vi "Window Plots.vi"() -> ()   [LabVIEW 2009]
uses:
  <vilib>/Analysis/4window.llb/Force Window (DBL).vi
  <vilib>/Analysis/4window.llb/Kaiser-Bessel Window (DBL).vi
  <vilib>/Analysis/4window.llb/Hamming Window (DBL).vi
  <vilib>/Analysis/4window.llb/Hanning Window (DBL).vi
  <vilib>/Analysis/4window.llb/Triangle Window (DBL).vi
  <vilib>/Analysis/4window.llb/Exponential Window (DBL).vi
  <vilib>/Analysis/NI_AALBase.lvlib
  <vilib>/Analysis/NI_AALPro.lvlib
panel:
  in  "beta (Kaiser-Bessel)":dbl=10.0 format="%.2f"
  in  "final value (exponential)":dbl=0.1 min=0.0 max=1.01 step=0.05 format="%.2f"
  out "Window":dbl[](graph)=[1.0, 0.9820327790631257, 0.9643883791544459, 0.9470610000772238, 0.9300449458481391, 0.9133346228248623, 0.8969245378672713, 0.8808092965317061, 0.8649836012976682, 0.8494422498263797, 0.8341801332506336, 0.8191922344953683, 0.8044736266284181, 0.7900194712408969, 0.775825016856679, 0.7618855973704608, 0.7481966305138833, 0.7347536163492154, 0.7215521357901017, 0.7085878491488874, 0.6958564947100447, 0.6833538873292304, 0.6710759170575142, 0.6590185477903263, 0.6471778159406794, 0.6355498291362295, 0.6241307649397461, 0.6129168695925733, 0.6019044567806661, 0.5910899064227986, 0.5804696634805439, 0.5700402367896358, 0.5597981979123283, 0.5497401800103734, 0.5398628767382501, 0.5301630411562773, 0.5206374846632573, 0.5112830759482941, 0.5020967399614464, 0.4930754569028748, 0.48421626123015066, 0.4755162406834013, 0.46697253532797073, 0.45858233661428077, 0.4503428864545839, 0.44225147631630474, 0.43430544633167084, 0.4265021844233419, 0.41883912544574825, 0.4113137503418573, 0.40392358531509076, 0.39666620101612016, 0.389539211744273, 0.38254027466328777, 0.37566708903115986, 0.3689173954438246, 0.3622889750924292, 0.3557796490339497, 0.3493872774749131, 0.3431097590679883, 0.336945030221216, 0.3308910644196496, 0.32494587155918425, 0.31910749729235516, 0.31337402238589035, 0.3077435620898061, 0.3022142655178378, 0.2967843150390036, 0.29145192568009887, 0.28621534453892705, 0.2810728502080725, 0.27602275220902706, 0.27106339043648336, 0.2661931346126128, 0.26141038375114883, 0.2567135656310988, 0.2521011362799121, 0.24757157946593383, 0.24312340619997844, 0.23875515424585797, 0.23446538763970512, 0.23025269621793265, 0.22611569515367402, 0.222053024501553, 0.21806334875063244, 0.21414535638539514, 0.21029775945461304, 0.20651929314796233, 0.20280871538024578, 0.19916480638308523, 0.19558636830395051, 0.19207222481239256, 0.1886212207133513, 0.18523222156741156, 0.1819041133178818, 0.17863580192457318, 0.17542621300415864, 0.17227429147699375, 0.1691790012202831, 0.16613932472747853, 0.1631542627737968, 0.16022283408774715, 0.15734407502856043, 0.15451703926941412, 0.1517407974863489, 0.14901443705277412, 0.14633706173946298, 0.14370779141993703, 0.14112576178114475, 0.1385901240393382, 0.1361000446610546, 0.13365470508911098, 0.13125330147352218, 0.12889504440725325, 0.12657915866671993, 0.12430488295695132, 0.12207146966133149, 0.1198781845958374, 0.11772430676769262, 0.11560912813835714, 0.11353195339077587, 0.1114920997008089, 0.10948889651276847, 0.10752168531898901, 0.10558981944335767, 0.10369266382873421, 0.10182959482819032, 0.09999999999999984]
  in  "stop":bool
  out "?":string="Exponential"
  out "Original Sine Wave":dbl[](graph)=[0.0, 0.47139673682599764, 0.8314696123025452, 0.9951847266721968, 0.9238795325112867, 0.6343932841636455, 0.19509032201612816, -0.29028467725446255, -0.7071067811865477, -0.9569403357322088, -0.9807852804032304, -0.7730104533627369, -0.38268343236508956, 0.09801714032956091, 0.5555702330196025, 0.8819212643483553, 1.0, 0.8819212643483552, 0.5555702330196023, 0.09801714032956063, -0.38268343236508984, -0.7730104533627371, -0.9807852804032305, -0.9569403357322087, -0.7071067811865472, -0.2902846772544619, 0.19509032201612886, 0.634393284163646, 0.9238795325112871, 0.9951847266721968, 0.8314696123025447, 0.4713967368259967, -1.1640536624890618e-15, -0.47139673682599875, -0.831469612302545, -0.9951847266721967, -0.9238795325112882, -0.6343932841636497, -0.1950903220161353, 0.2902846772544539, 0.70710678118654, 0.9569403357322053, 0.9807852804032332, 0.7730104533627469, 0.3826834323651057, -0.09801714032954173, -0.5555702330195851, -0.8819212643483445, -1.0, -0.8819212643483672, -0.5555702330196249, -0.09801714032958952, 0.38268343236506136, 0.7730104533627163, 0.9807852804032238, 0.9569403357322193, 0.707106781186574, 0.29028467725449986, -0.1950903220160882, -0.6343932841636126, -0.9238795325112699, -0.9951847266722014, -0.8314696123025717, -0.4713967368260411, -5.096259785702939e-14, 0.47139673682595123, 0.831469612302515, 0.9951847266721917, 0.9238795325113062, 0.6343932841636831, 0.19509032201617424, -0.2902846772544193, -0.707106781186517, -0.956940335732197, -0.9807852804032381, -0.7730104533627608, -0.3826834323651227, 0.09801714032952698, 0.5555702330195756, 0.8819212643483408, 1.0, 0.8819212643483675, 0.5555702330196225, 0.09801714032958306, -0.38268343236507063, -0.773010453362725, -0.9807852804032271, -0.9569403357322133, -0.7071067811865569, -0.29028467725447327, 0.19509032201611895, 0.6343932841636396, 0.9238795325112845, 0.9951847266721973, 0.8314696123025463, 0.4713967368259978, -1.715804148066935e-15, -0.4713967368260008, -0.8314696123025482, -0.9951847266721976, -0.9238795325112832, -0.6343932841636369, -0.1950903220161156, 0.29028467725447654, 0.7071067811865593, 0.9569403357322143, 0.9807852804032264, 0.7730104533627228, 0.38268343236506747, -0.09801714032958649, -0.5555702330196254, -0.881921264348369, -1.0, -0.8819212643483393, -0.5555702330195729, -0.09801714032952356, 0.38268343236512586, 0.773010453362763, 0.9807852804032388, 0.956940335732196, 0.7071067811865146, 0.29028467725441603, -0.1950903220161776, -0.6343932841636858, -0.9238795325113074, -0.9951847266721914, -0.8314696123025132, -0.4713967368259451]
  out "Windowed Sine Wave":dbl[](graph)=[0.0, 0.46292704750652336, 0.801859631724627, 0.9425006425037493, 0.8592494897846639, 0.5794133509142289, 0.1749812969166929, -0.25568544236643653, -0.6116357700927423, -0.8128655517339787, -0.8181515958970268, -0.6332441605784981, -0.3078587286853546, 0.0774354493757045, 0.43102528539750223, 0.6719231093217588, 0.7481966305138833, 0.6479948383152263, 0.4008728882166985, 0.06945375464584803, -0.2662927518291799, -0.5282396982515571, -0.6581813814831091, -0.6306414303762274, -0.4576238222851535, -0.18449037702993876, 0.1217618719122679, 0.3888303458201337, 0.556087208146982, 0.5882436469620672, 0.48264288604755634, 0.2687151074821528, -6.516351425346225e-16, -0.2591457269590272, -0.4488795768180894, -0.5276101612048104, -0.48100631593854315, -0.32435454968813104, -0.09795421468233033, 0.1431322498691434, 0.3423926018766326, 0.4550406710056902, 0.4579997890022525, 0.35448893993035296, 0.17233876152964925, -0.04334822501504224, -0.24128717802016128, -0.3761413457339645, -0.41883912544574825, -0.3627463427453594, -0.22440792041562735, -0.03888008668900222, 0.14907020259107878, 0.2957076311469661, 0.368448751253689, 0.3530319362534694, 0.2561769910369905, 0.10327738059353932, -0.06816207647090515, -0.21766652688372698, -0.3112966170027727, -0.3292977335027428, -0.27018261784463615, -0.15042623292034096, -1.5970354281691857e-14, 0.1450693109483291, 0.25128197818240594, 0.2953552174426844, 0.2692664688468497, 0.18157309240009, 0.05483459285709677, -0.08012517553987399, -0.19167076150904586, -0.2547309476057996, -0.25638745652768863, -0.19844226975286655, -0.09647492813474431, 0.024266258246115075, 0.13507212743503497, 0.2105632475021902, 0.23446538763970512, 0.20306474896813972, 0.1256231494459206, 0.021765002463177068, -0.08344923077291345, -0.16553659902499662, -0.20625694697486305, -0.19762664172019045, -0.14340741792910613, -0.05781449154136355, 0.038157007574380945, 0.12184932949535061, 0.1742632852143588, 0.18434027779144835, 0.15124774257665763, 0.0842083341075391, -3.009970239522091e-16, -0.08120953884126618, -0.14066719855436113, -0.1653393184684192, -0.15073488401867846, -0.10164428991493142, -0.030696306264649705, 0.04485392887463916, 0.10729694688525371, 0.1425979254222286, 0.14352523613152346, 0.11108762499728111, 0.05400649091354333, -0.013584207636258611, -0.07561313352632353, -0.11787292649829716, -0.13125330147352218, -0.11367528053188013, -0.07032361267589107, -0.012184009156436498, 0.046714729003853664, 0.09266708982273326, 0.1154622672234283, 0.11063103789442594, 0.08027921412396893, 0.03236444817806649, -0.021360224077871946, -0.06821103506832779, -0.09755227302528263, -0.10319335531031028, -0.0846682137327174, -0.04713967368259443]
  in  "Window Selector":T1(ring)=enum."Exponential"
  out "Window (time domain)":dbl[][](graph)=[[1.0, 1.0, 1.0, 1.0, 1.0, 1.0, 1.0, 1.0, 1.0, 1.0, 1.0, 1.0, 1.0, 1.0, 1.0, 1.0, 1.0, 1.0, 1.0, 1.0], [0.0, 0.09999999999999998, 0.19999999999999996, 0.30000000000000004, 0.4, 0.5, 0.6, 0.7, 0.8, 0.9, 1.0, 0.9, 0.8, 0.7, 0.6, 0.5, 0.4, 0.30000000000000004, 0.19999999999999996, 0.09999999999999998], [0.0, 0.024471741852423214, 0.09549150281252629, 0.20610737385376343, 0.3454915028125263, 0.5, 0.6545084971874737, 0.7938926261462366, 0.9045084971874737, 0.9755282581475768, 1.0, 0.9755282581475768, 0.9045084971874737, 0.7938926261462366, 0.6545084971874737, 0.5, 0.3454915028125263, 0.20610737385376343, 0.09549150281252629, 0.024471741852423214], [0.08, 0.10251400250422936, 0.16785218258752418, 0.26961878394546235, 0.3978521825875242, 0.54, 0.6821478174124758, 0.8103812160545376, 0.9121478174124759, 0.9774859974957707, 1.0, 0.9774859974957707, 0.9121478174124759, 0.8103812160545376, 0.6821478174124758, 0.54, 0.3978521825875242, 0.26961878394546235, 0.16785218258752418, 0.10251400250422936], [1.0, 0.8858667904100826, 0.7847599703514613, 0.6951927961775606, 0.6158482110660264, 0.5455594781168519, 0.4832930238571753, 0.4281332398719394, 0.37926901907322497, 0.3359818286283782, 0.2976351441631318, 0.26366508987303583, 0.23357214690901223, 0.20691380811147897, 0.18329807108324359, 0.16237767391887217, 0.14384498882876628, 0.12742749857031338, 0.1128837891684689, 0.1], [0.0003551493747240969, 0.0054848601297265, 0.02387825759759729, 0.06825719363378314, 0.15184912835301753, 0.28205962082270336, 0.45385517966505423, 0.6463901001143227, 0.825681302169712, 0.9535699613018814, 1.0, 0.9535699613018814, 0.825681302169712, 0.6463901001143227, 0.45385517966505423, 0.28205962082270336, 0.15184912835301753, 0.06825719363378314, 0.02387825759759729, 0.0054848601297265]]
  # "Rectangular"
  # "Triangle"
  # "Hanning"
  # "Hamming"
  # "Exponential"
  # "Kaiser-Bessel"
  # "="
  # "X"
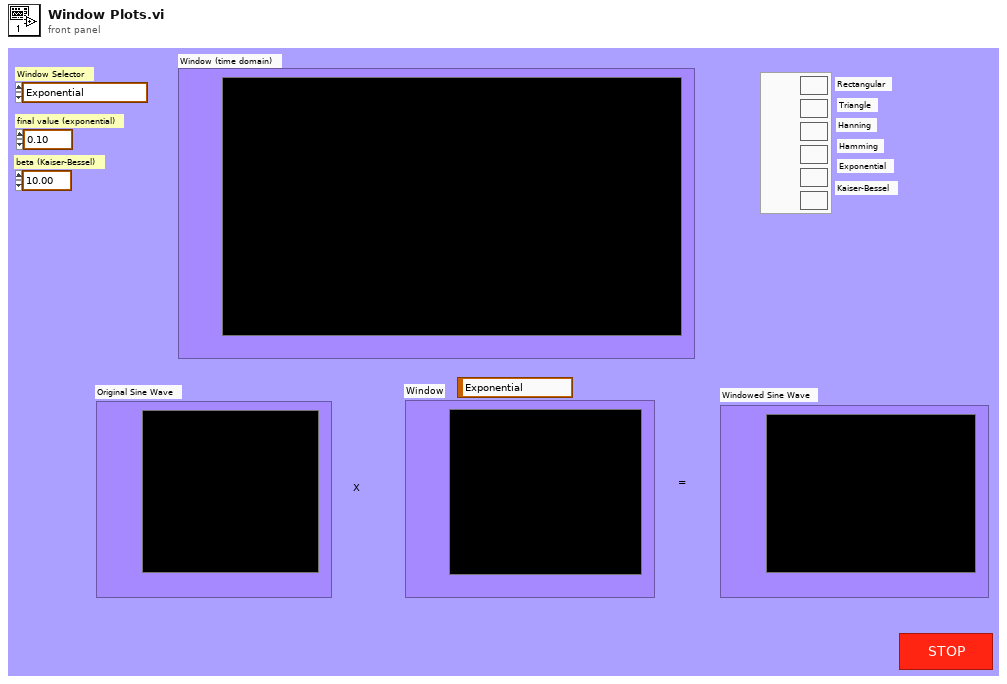
[diagram p1: front panel]
types:
  T1 = enum16{"Hamming", "Hanning", "Triangle", "Rectangular (None)", "Exponential", "Kaiser-Bessel"}
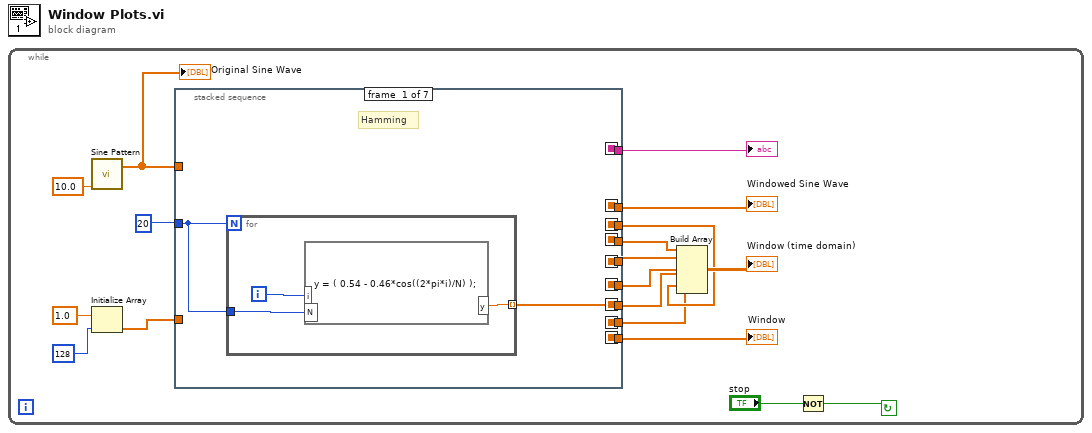
[diagram p0: block diagram]
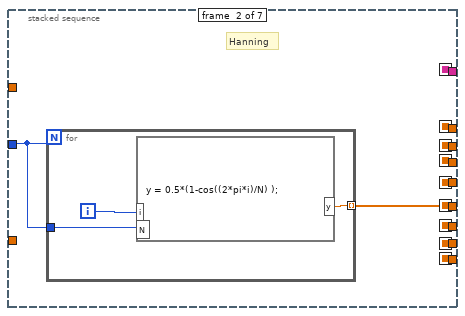
[diagram p2: hidden frame]
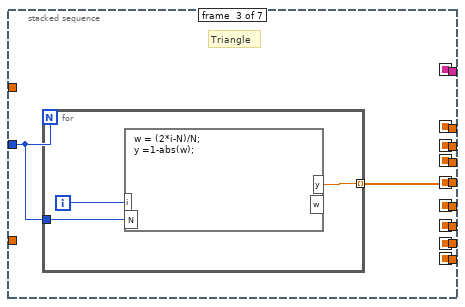
[diagram p3: hidden frame]
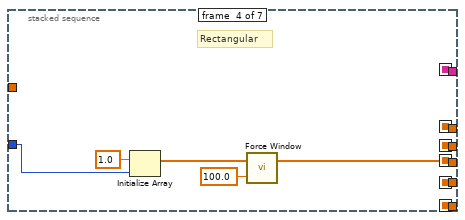
[diagram p4: hidden frame]
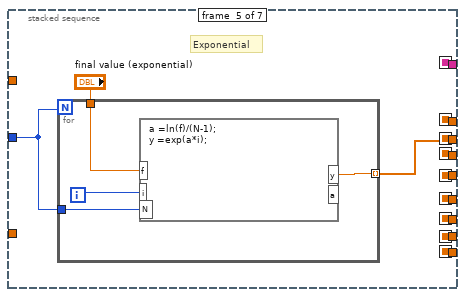
[diagram p5: hidden frame]
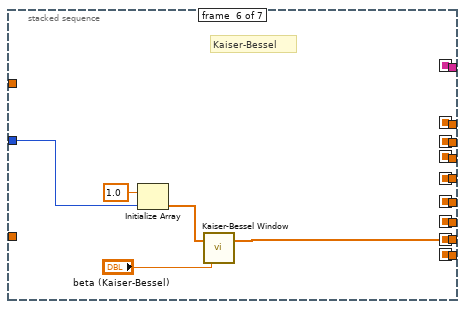
[diagram p6: hidden frame]
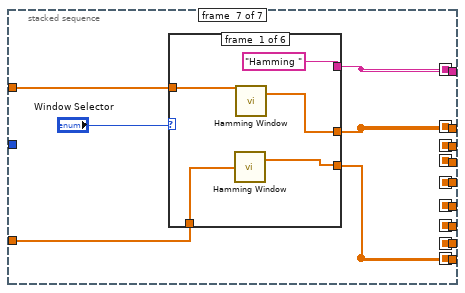
[diagram p7: hidden frame]
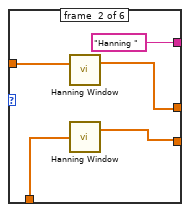
[diagram p8: hidden frame]
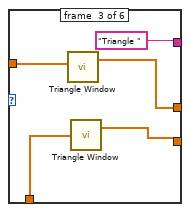
[diagram p9: hidden frame]
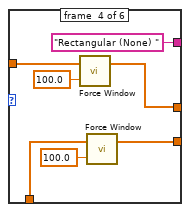
[diagram p10: hidden frame]
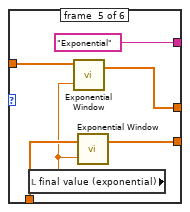
[diagram p11: hidden frame]
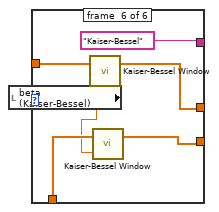
[diagram p12: hidden frame]
diagram:
  n1 = while {
    stop <- w9 continue-if-true
    n2 = call <vilib>:"Sine Pattern.vi"("cycles"=10.0) -> ("Sinusoidal Pattern"=w7:dbl[])  [unwired: 3 in, 1 out]
    "Original Sine Wave" <- w7
    n3 = Initialize Array(1.0, 128) -> (w4:dbl[])
    n4 = stacked-sequence {
      seq-local: [w19 _ _ _ _ _ _] -> [_ _ _ _ _ _ w58]
      seq-local: [_ w24 _ _ _ _ _] -> [_ _ _ _ _ _ w59]
      seq-local: [_ _ w29 _ _ _ _] -> [_ _ _ _ _ _ w60]
      seq-local: [_ _ _ w35 _ _ _] -> [_ _ _ _ _ _ _]
      seq-local: [_ _ _ _ _ _ w56] -> [_ _ _ _ _ _ _]
      seq-local: [_ _ _ _ _ _ w55] -> [_ _ _ _ _ _ _]
      seq-local: [_ _ _ _ _ _ w52] -> [_ _ _ _ _ _ _]
      seq-local: [_ _ _ _ w40 _ _] -> [_ _ _ _ _ _ w51]
      seq-local: [_ _ _ _ _ w49 _] -> [_ _ _ _ _ _ _]
      tunnel: 20 -> [w20 w25 w30 w34 w41 w47 _]
      tunnel: [_ _ _ _ _ _ w60] -> w13
      tunnel: [_ _ _ _ _ _ w59] -> w15
      tunnel: [_ _ _ _ _ _ w58] -> w12
      tunnel: [_ _ _ w35 _ _ _] -> w14
      tunnel: [_ _ _ _ _ _ w56] -> w8
      tunnel: [_ _ _ _ _ _ w55] -> w18
      tunnel: w7 -> [_ _ _ _ _ _ w54]
      tunnel: w4 -> [_ _ _ _ _ _ w53]
      tunnel: [_ _ _ _ _ _ w52] -> w3
      tunnel: [_ _ _ _ _ _ w51] -> w2
      tunnel: [_ _ _ _ _ w49 _] -> w1
      frame #0 {
        # "Hamming"
        n5 = for {
          N: w20 -> [_]
          tunnel: w20 -> [w23]
          tunnel: [w22] -> w19 mode=indexing
          i -> [w21]
          n6 = formula code="y = ( 0.54 - 0.46*cos((2*pi*i)/N) );"("i"=w21, "N"=w23) -> ("y"=w22:dbl)
        }
      }
      frame #1 {
        # "Hanning"
        n7 = for {
          N: w25 -> [_]
          tunnel: [w28] -> w24 mode=indexing
          tunnel: w25 -> [w27]
          i -> [w26]
          n8 = formula code="y = 0.5*(1-cos((2*pi*i)/N) );"("i"=w26, "N"=w27) -> ("y"=w28:dbl)
        }
      }
      frame #2 {
        # "Triangle"
        n9 = for {
          N: w30 -> [_]
          tunnel: [w33] -> w29 mode=indexing
          tunnel: w30 -> [w32]
          i -> [w31]
          n10 = formula code="w = (2*i-N)/N;\ny =1-abs(w);"("i"=w31, "N"=w32) -> ("y"=w33:dbl)  [unwired: 1 out]
        }
      }
      frame #3 {
        # "Rectangular"
        n11 = Initialize Array(1.0, w34) -> (w36:dbl[])
        n12 = call-poly <vilib>:"Force Window.vi"("duty cycle(%)"=100.0, "X"=w36) -> ("Windowed X"=w35:dbl[])  [unwired: 1 out]
      }
      frame #4 {
        # "Exponential"
        n13 = for {
          N: w41 -> [_]
          tunnel: w41 -> [w45]
          tunnel: [w43] -> w40 mode=indexing
          tunnel: "final value (exponential)" -> [w42]
          i -> [w44]
          n14 = formula code="a =ln(f)/(N-1);\ny =exp(a*i);"("i"=w44, "N"=w45, "f"=w42) -> ("y"=w43:dbl)  [unwired: 1 out]
        }
      }
      frame #5 {
        # "Kaiser-Bessel"
        n15 = Initialize Array(1.0, w47) -> (w46:dbl[])
        n16 = call-poly <vilib>:"Kaiser-Bessel Window.vi"("beta"="beta (Kaiser-Bessel)", "X"=w46) -> ("Windowed X"=w49:dbl[])  [unwired: 1 out]
      }
      frame #6 {
        n17 = case shown="\"Exponential\"" "Window Selector" {
          tunnel: [w65 w70 w75 w82 w85 w93] -> w56
          tunnel: ["Hamming " "Hanning " "Triangle " "Rectangular (None) " "Exponential" "Kaiser-Bessel"] -> w55
          tunnel: w54 -> [w63 w68 w73 w79 w88 w94]
          tunnel: w53 -> [w62 w67 w72 w77 w87 w92]
          tunnel: [w61 w66 w71 w76 w86 w91] -> w52
          frame #0 {
            n18 = call-poly <vilib>:"Hamming Window.vi"("X"=w62) -> ("Windowed X"=w61:dbl[])  [unwired: 1 out]
            n19 = call-poly <vilib>:"Hamming Window.vi"("X"=w63) -> ("Windowed X"=w65:dbl[])  [unwired: 1 out]
          }
          frame #1 {
            n20 = call-poly <vilib>:"Hanning Window.vi"("X"=w68) -> ("Windowed X"=w70:dbl[])  [unwired: 1 out]
            n21 = call-poly <vilib>:"Hanning Window.vi"("X"=w67) -> ("Windowed X"=w66:dbl[])  [unwired: 1 out]
          }
          frame #2 {
            n22 = call-poly <vilib>:"Triangle Window.vi"("X"=w73) -> ("Windowed X"=w75:dbl[])  [unwired: 1 out]
            n23 = call-poly <vilib>:"Triangle Window.vi"("X"=w72) -> ("Windowed X"=w71:dbl[])  [unwired: 1 out]
          }
          frame #3 {
            n24 = call-poly <vilib>:"Force Window.vi"("duty cycle(%)"=100.0, "X"=w79) -> ("Windowed X"=w82:dbl[])  [unwired: 1 out]
            n25 = call-poly <vilib>:"Force Window.vi"("duty cycle(%)"=100.0, "X"=w77) -> ("Windowed X"=w76:dbl[])  [unwired: 1 out]
          }
          frame #4 {
            n26 = local read "final value (exponential)"() -> (w83:dbl)
            n27 = call-poly <vilib>:"Exponential Window.vi"("final value"=w83, "X"=w88) -> ("Windowed X"=w85:dbl[])  [unwired: 1 out]
            n28 = call-poly <vilib>:"Exponential Window.vi"("final value"=w83, "X"=w87) -> ("Windowed X"=w86:dbl[])  [unwired: 1 out]
          }
          frame #5 {
            n29 = local read "beta (Kaiser-Bessel)"() -> (w89:dbl)
            n30 = call-poly <vilib>:"Kaiser-Bessel Window.vi"("beta"=w89, "X"=w94) -> ("Windowed X"=w93:dbl[])  [unwired: 1 out]
            n31 = call-poly <vilib>:"Kaiser-Bessel Window.vi"("beta"=w89, "X"=w92) -> ("Windowed X"=w91:dbl[])  [unwired: 1 out]
          }
        }
      }
    }
    "?" <- w18
    "Windowed Sine Wave" <- w8
    "Window" <- w3
    n32 = Build Array(w14, w13, w15, w12, w2, w1) -> (→"Window (time domain)":dbl[][])
    n33 = Not(x="stop") -> (.not. x?=w9:bool)
  }
